vi "Periodic Tasks.vi"(8 "error in":errorcluster) -> ()   [LabVIEW 2017]
doc: "This VI runs in parallel to other tasks. It can contain as many user-defined periodic loops as you need. These can carry out PID or other sorts of timed response."
uses:
  <vilib>/Rock Robotics/WPI/ThirdParty/Phoenix-LabVIEW/Motor Controller/Controls/CTRE_Phoenix_MotorControl_ControlMode.ctl
panel:
  in  "Numeric":dbl
  out "Position (Raw Sensor Units)":i32
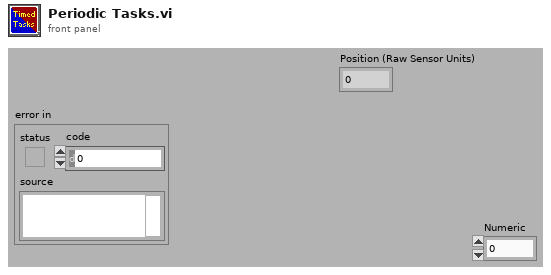
[diagram p1: front panel]
types:
  T1 = typedef "WPI_MotorControlDeviceRef.ctl" = cluster{"DeviceStatus":errorcluster, "Type":T2, "PWM":cluster{"PWM Channel":T3, "DeadBand":T4}, "CAN":cluster{"Device Number":u8, "SetOutput VI Ref":variant, "GetOutput VI Ref":variant, "Enable VI Ref":variant, "Disable VI Ref":variant, "Data":variant}, "Invert":bool, "DIO PWM":cluster{"PWM \"Enable\" Channel":T3, "DIOChannel":T5, "PWM Rate":dbl}}
  T2 = typedef "WPI_MotorControlType.ctl" = enum16{"PWM", "CAN", "DIO PWM"}
  T3 = typedef "FPGA_DIOPWMChannel.ctl" = enum8{"PWM 0", "PWM 1", "PWM 2", "PWM 3", "PWM 4", "PWM 5", "PWM 6", "PWM 7", "PWM 8", "PWM 9", "PWM MXP 0", "PWM MXP 1", "PWM MXP 2", "PWM MXP 3", "PWM MXP 4", "PWM MXP 5", "PWM MXP 6", "PWM MXP 7", "PWM MXP 8", "PWM MXP 9", "Invalid"}
  T4 = typedef "WPI_PWMDeadband.ctl" = cluster{"Name":string, "maxPositivePwm":i32, "minPositivePwm":i32, "centerPwm":i32, "maxNegativePwm":i32, "minNegativePwm":i32, "angularRange":u16}
  T5 = typedef "FPGA_DIOChannel.ctl" = enum8{"DIO 0", "DIO 1", "DIO 2", "DIO 3", "DIO 4", "DIO 5", "DIO 6", "DIO 7", "DIO 8", "DIO 9", "DIO MXP 0", "DIO MXP 1", "DIO MXP 2", "DIO MXP 3", "DIO MXP 4", "DIO MXP 5", "DIO MXP 6", "DIO MXP 7", "DIO MXP 8", "DIO MXP 9", "DIO MXP 10", "DIO MXP 11", "DIO MXP 12", "DIO MXP 13", "DIO MXP 14", "DIO MXP 15", "SPI Port CS1", "SPI Port CS2", "SPI Port CS3", "SPI Port MISO", "SPI Port MOSI", "Invalid"}
  T6 = typedef "CTRE_Phoenix_MotorControl_ControlMode.ctl" = u16
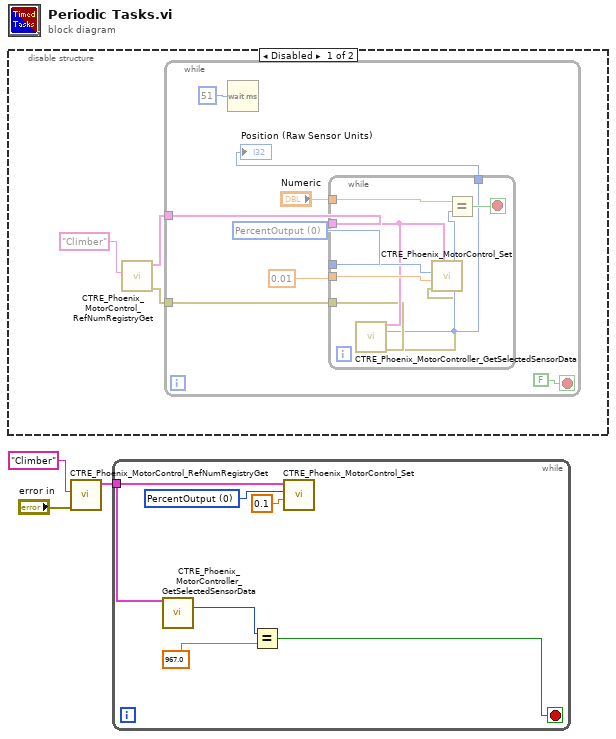
[diagram p0: block diagram]
diagram:
  n1 = disable-structure shown="Disabled" {
    frame Disabled {
      n2 = call "CTRE_Phoenix_MotorControl_RefNumRegistryGet.vi"("refnum name"="Climber") -> ("error out"=w4:errorcluster, "PhoenixMotorControlDevRef"=w5:T1)  [unwired: 9 in]
      n3 = while {
        tunnel: w5 -> [w9]
        tunnel: w4 -> [w8]
        stop <- FALSE stop-if-true
        w10 = T6 0 items=["PercentOutput"=0, "Position"=1, "Velocity"=2, "Current"=3, "Follower"=5, "MotionProfile"=6, "MotionMagic"=7, "MotionMagicArc"=8, "MotionProfileArc"=10, "Disabled"=15] ("Control Mode")
        n4 = Wait (ms)(milliseconds to wait=u32 51) -> ()  [unwired: 1 out]
        n5 = while {
          tunnel: "Numeric" -> [w22]
          tunnel: 0.01 ("Slide") -> [w20]
          tunnel: w10 -> [w19]
          tunnel: w9 -> [w18]
          tunnel: w8 -> [w17]
          tunnel: [w16] -> w7
          stop <- w21 stop-if-true
          n6 = call "CTRE_Phoenix_MotorController_GetSelectedSensorData.vi"("PhoenixMotorControlDevRef"=w18, "error in"=w17) -> ("Position (Raw Sensor Units)"=w16:i32, "error out"=w15:errorcluster)  [unwired: 10 in, 2 out]
          n7 = call "CTRE_Phoenix_MotorControl_Set.vi"("error in (no error)"=w15, "Output"=w20, "Control Mode"=w19, "PhoenixMotorControlDevRef"=w18) -> ()  [unwired: 6 in, 2 out]
          n8 = Equal?(x=w22, y=w16) -> (x = y?=w21:bool)
        }
        "Position (Raw Sensor Units)" <- w7
      }
    }
    frame Enabled {
    }
  }
  n9 = call "CTRE_Phoenix_MotorControl_RefNumRegistryGet.vi"("error in (no error)"="error in", "refnum name"="Climber") -> ("PhoenixMotorControlDevRef"=w3:T1)  [unwired: 8 in, 1 out]
  n10 = while {
    tunnel: w3 -> [w26]
    stop <- w23 stop-if-true
    w28 = T6 0 items=["PercentOutput"=0, "Position"=1, "Velocity"=2, "Current"=3, "Follower"=5, "MotionProfile"=6, "MotionMagic"=7, "MotionMagicArc"=8, "MotionProfileArc"=10, "Disabled"=15] ("Control Mode")
    n11 = call "CTRE_Phoenix_MotorController_GetSelectedSensorData.vi"("PhoenixMotorControlDevRef"=w26) -> ("Position (Raw Sensor Units)"=w25:i32)  [unwired: 11 in, 3 out]
    n12 = Equal?(x=w25, y=967.0) -> (x = y?=w23:bool)
    n13 = call "CTRE_Phoenix_MotorControl_Set.vi"("Output"=0.1, "Control Mode"=w28, "PhoenixMotorControlDevRef"=w26) -> ()  [unwired: 7 in, 2 out]
  }
